vi "Global communication output.vi"() -> ()   [LabVIEW 2016]
panel:
  in  "Fault control":bool[](array[boolean])
  in  "Gen Control from MGCC":dbl[](array[numeric])
  in  "BESS2 Control from MGCC":dbl[](array[numeric])
  in  "PV Control from MGCC":dbl[](array[numeric])
  in  "BESS1 Control from MGCC":dbl[](array[numeric])
  in  "comm_matrix":dbl[][](array[numeric])
  in  "LC2 Control":dbl[](array[numeric])
  in  "LC1 Control":dbl[](array[numeric])
  in  "Gen Control":dbl[](array[numeric])
  in  "BESS2 Control":dbl[](array[numeric])
  in  "PV Temp":dbl[](array[numeric])
  in  "PV Control":dbl[](array[numeric])
  in  "BESS1 Control":dbl[](array[numeric])
  in  "IntellRupter Control":bool[](array[boolean])
  in  "Matrix output":bool
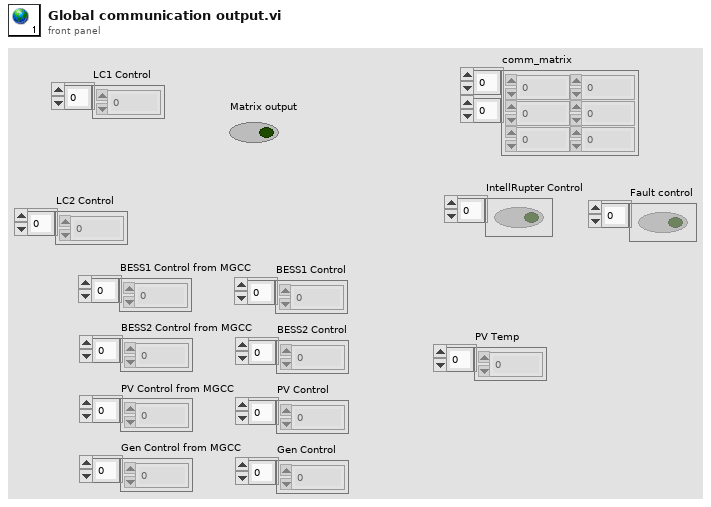
[diagram p1: front panel]
diagram:
